vi "MICSD CW Carrier.vi"(6 "400MHz Channel":u8, 8 "error in (no error)":errorcluster, 9 "TX Mode (Off)":bool, 10 "Frequency Range":enum16{"2.45GHz", "400MHz"}(ring), 11 "VISA Resource Name":refnum<visa-resource-name>) -> (0 "error out":errorcluster, 3 "dup VISA Resource Name":refnum<visa-resource-name>)   [LabVIEW 2010]
uses:
  <vilib>/Instr/_visa.llb/VISA Configure Serial Port (Instr).vi
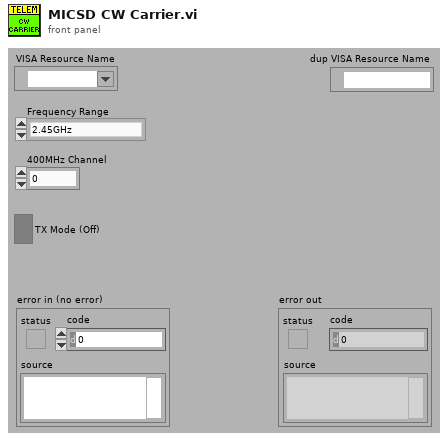
[diagram p1: front panel]
types:
  T1 = cluster{"Command Token":u8, "Length":u16, "Pack Data":u8[]}
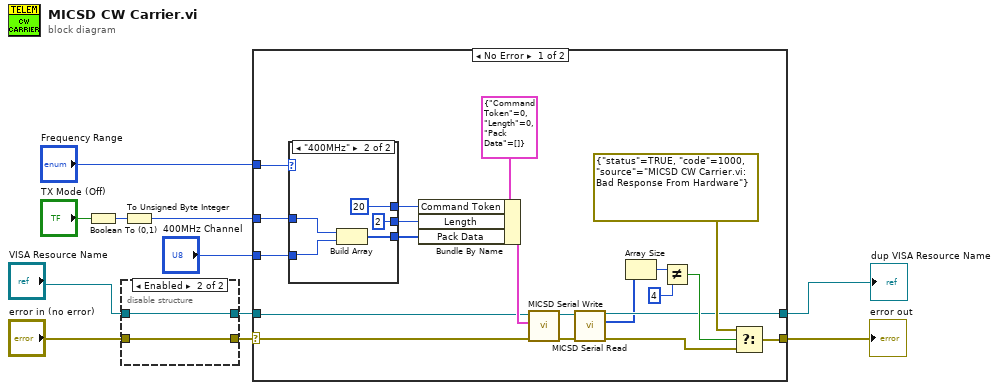
[diagram p0: block diagram]
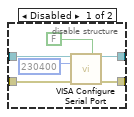
[diagram p2: hidden frame]
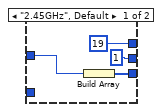
[diagram p3: hidden frame]
diagram:
  n1 = Boolean To (0,1)(Boolean="TX Mode (Off)") -> (0, 1=w3:i16)
  n2 = disable-structure shown="Enabled" {
    disable-tunnel: [w15 w18] -> w10
    disable-tunnel: "error in (no error)" -> [w14 w18]
    disable-tunnel: "VISA Resource Name" -> [w13 w19]
    disable-tunnel: [w12 w19] -> w7
    frame Disabled {
      n3 = call-poly "VISA Configure Serial Port"("VISA resource name"=w13, "Enable Termination\nChar (T)"=FALSE ("Enable Termination\nChar (T)"), "baud rate (9600)"=u32 230400, "error in (no error)"=w14) -> ("VISA resource name out"=w12:refnum<visa-resource-name>, "error out"=w15:errorcluster)  [unwired: 10 in]
    }
    frame Enabled {
    }
  }
  n4 = To Unsigned Byte Integer(number=w3) -> (unsigned 8bit integer=w2:u8)
  n5 = case shown="No Error" w10 {
    selector: w10 -> [w37 w50]
    tunnel: [w20 w50] -> w1
    tunnel: w7 -> [w36 w49]
    tunnel: [w23 w49] -> w11
    tunnel: "Frequency Range" -> [w35 _]
    tunnel: w2 -> [w29 _]
    tunnel: "400MHz Channel" -> [w28 _]
    frame No Error {
      n6 = case shown="\"400MHz\"" w35 {
        tunnel: [u16 19 ("Length") u16 20 ("Length")] -> w34
        tunnel: [u16 1 ("Length") u16 2 ("Length")] -> w31
        tunnel: [w41 w46] -> w30
        tunnel: w29 -> [w40 w44]
        tunnel: w28 -> [_ w45]
        frame "2.45GHz", Default {
          n7 = Build Array(w40) -> (w41:u8[])
        }
        frame "400MHz" {
          n8 = Build Array(w44, w45) -> (w46:u8[])
        }
      }
      n9 = Bundle By Name(cluster=T1 {"Command Token"=0, "Length"=0, "Pack Data"=[]} ("Write Data"), "Command Token"=w34, "Length"=w31, "Pack Data"=w30) -> (w39:T1)
      n10 = call "MICSD Serial Write.vi"("error in (no error)"=w37, "Write Data"=w39, "VISA Resource Name"=w36) -> ("error out"=w32:errorcluster, "DUP Visa Resource Name"=w33:refnum<visa-resource-name>)  [unwired: 7 in]
      n11 = call "MICSD Serial Read.vi"("error in (no error)"=w32, "VISA Resource Name"=w33) -> ("error out"=w21:errorcluster, "Read Data"=w22:u8[], "DUP Visa Resource Name"=w23:refnum<visa-resource-name>)  [unwired: 7 in]
      n12 = Array Size(array=w22) -> (size(s)=w26:i32)
      n13 = Not Equal?(x=w26, y=4) -> (x != y?=w25:bool)
      n14 = Select(t=errorcluster {"status"=TRUE, "code"=1000, "source"="MICSD CW Carrier.vi:  Bad Response From Hardware"} ("error IO"), s=w25, f=w21) -> (s? t:f=w20:errorcluster)
    }
    frame Error {
    }
  }
  "dup VISA Resource Name" <- w11
  "error out" <- w1
